vi "CSTK_BuildApplication_Manager_getEXEVersion.vi"(8 "错误输入（无错误）":errorcluster, 11 "EXE路径":path) -> (0 "错误输出":errorcluster, 3 "版本号":string)   [LabVIEW 2015, in "CSTK_BuildApplication_Manager.lvlib"]
doc: "该控件主要用作获取exe文件版本号\n\n作者: CLAN\n日期: 2021-10-12\n\nUID: [1001,1018,1062,1084,1108,1125,1157,1174,969]"
uses:
  CSTK_BuildApplication_Manager.lvlib
panel:
  # "输入"
  # "输入"
  # "过程"
  # "输出"
  # "注释"
  # "CLAN\n2021-10-12\n\n该控件主要用作获取exe文件版本号"
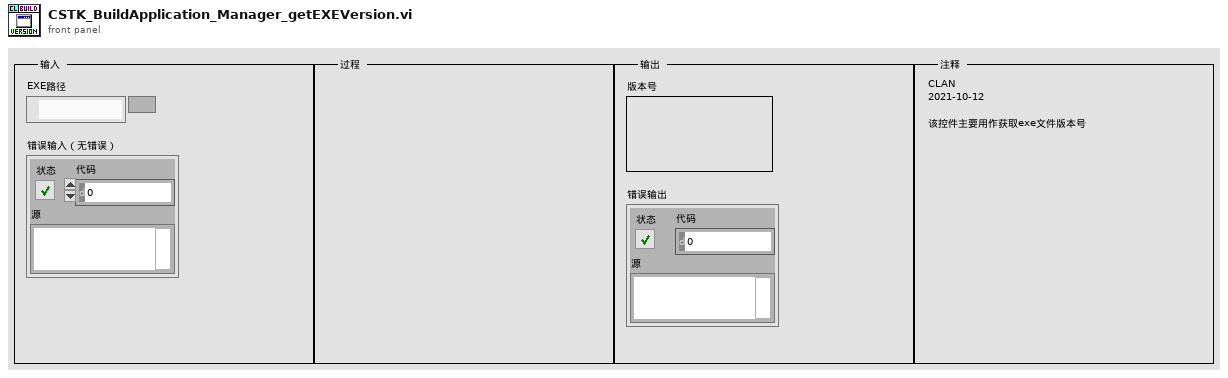
[diagram p1: front panel]
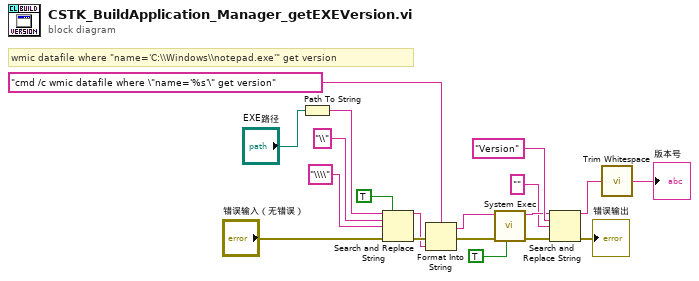
[diagram p0: block diagram]
diagram:
  # "wmic datafile where \"name='C:\\\\Windows\\\\notepad.exe'\" get version"
  n1 = Path To String(path="EXE路径") -> (string=w18:string)
  n2 = Search and Replace String(replace all?=TRUE ("替换全部？(F)"), input string=w18, search string="\\" ("搜索字符串"), replace string="\\\\" ("替换字符串(\"\")"), error in="错误输入（无错误）") -> (result string=w12:string, error out=w14:errorcluster)  [unwired: 3 in, 2 out]
  n3 = Format Into String(format string="cmd /c wmic datafile where \"name='%s'\" get version" ("格式字符串"), error in=w14, w12) -> (resulting string=w10:string, error out=w11:errorcluster)  [unwired: 1 in]
  n4 = call <vilib>:"System Exec.vi"("run minimized? (F)"=TRUE, "error in (no error)"=w11, "command line"=w10) -> ("error out"=w8:errorcluster, "standard output"=w6:string)  [unwired: 5 in, 2 out]
  n5 = Search and Replace String(input string=w6, search string="Version" ("搜索字符串"), replace string="" ("替换字符串(\"\")"), error in=w8) -> (result string=w4:string, error out=→"错误输出":errorcluster)  [unwired: 4 in, 2 out]
  n6 = call <vilib>:"Trim Whitespace.vi"("string"=w4) -> ("trimmed string"=→"版本号":string)  [unwired: 1 in]
